vi "test robot move.vi"() -> ()   [LabVIEW 2018]
panel:
  in  "stop":bool
  in  "stop 3":bool
  in  "stop 2":bool
  out "Battery Voltage Output":u16
  in  "speed":i32
  in  "distance":dbl
  in  "Enum":enum16{"forward", "backward", "left", "right"}(ring)
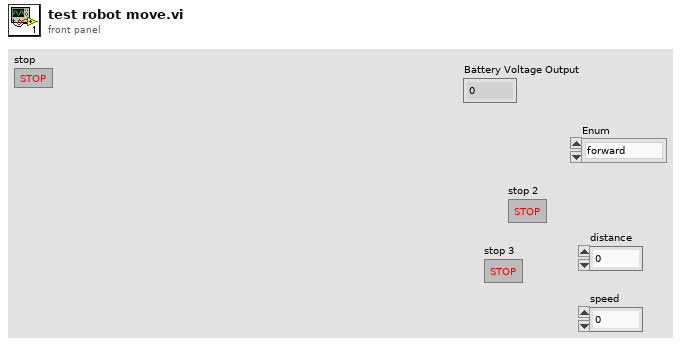
[diagram p1: front panel]
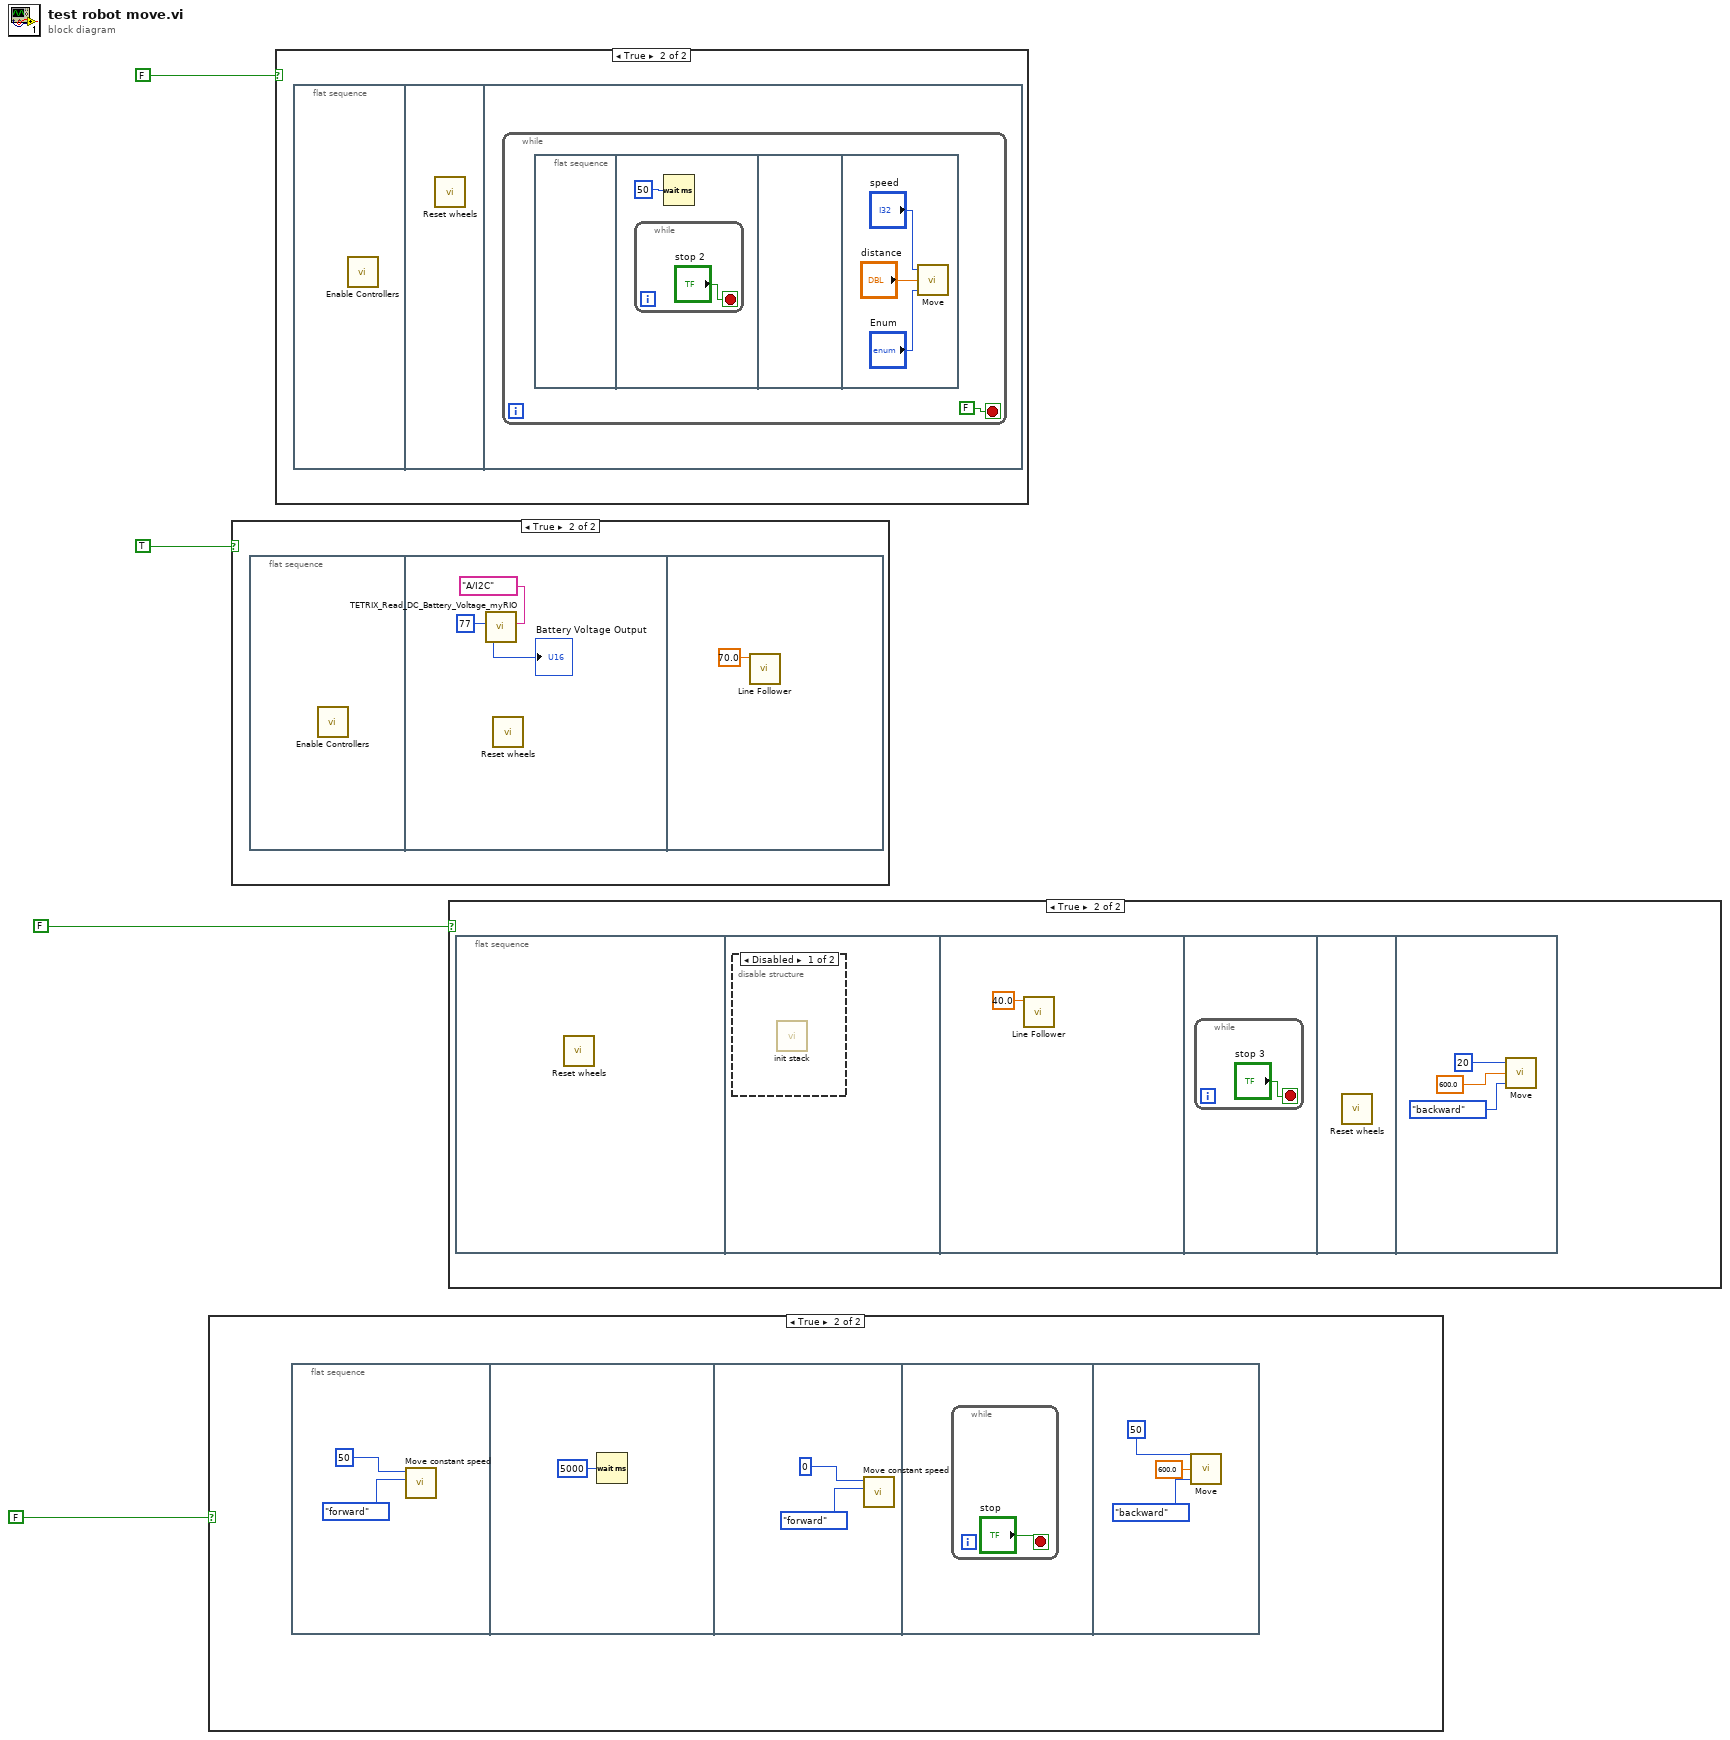
[diagram p0: block diagram]
diagram:
  n1 = case shown="True" FALSE {
    frame False {
    }
    frame True {
      n2 = flat-sequence {
        frame #0 {
          n3 = call "Move constant speed.vi"("Enum"=enum16{"forward", "backward", "left", "right"}."forward", "speed"=50) -> ()  [unwired: 10 in]
        }
        frame #1 {
          n4 = Wait (ms)(milliseconds to wait=u32 5000) -> ()  [unwired: 1 out]
        }
        frame #2 {
          n5 = call "Move constant speed.vi"("Enum"=enum16{"forward", "backward", "left", "right"}."forward", "speed"=0) -> ()  [unwired: 10 in]
        }
        frame #3 {
          n6 = while {
            stop <- "stop" stop-if-true
          }
        }
        frame #4 {
          n7 = call "Move.vi"("Enum"=enum16{"forward", "backward", "left", "right"}."backward", "distance"=600.0, "speed"=50) -> ()  [unwired: 1 in]
        }
      }
    }
  }
  n8 = case shown="True" TRUE {
    frame False {
    }
    frame True {
      n9 = flat-sequence {
        frame #0 {
          n10 = call "Enable Controllers.vi"() -> ()  [unwired: 12 in]
        }
        frame #1 {
          n11 = call <vilib>:"TETRIX_Read_DC_Battery_Voltage_myRIO.vi"("myRIO MXP Port A/B"=tag "A/I2C", "Controller ID#  (I2C Address)"=u8 77) -> ("Battery Voltage Output"=→"Battery Voltage Output":u16)  [unwired: 4 in, 1 out]
          n12 = call "Reset wheels.vi"() -> ()  [unwired: 12 in]
        }
        frame #2 {
          n13 = call "Line Follower.vi"("speed"=70.0) -> ()  [unwired: 11 in]
        }
      }
    }
  }
  n14 = case shown="True" FALSE {
    frame False {
    }
    frame True {
      n15 = flat-sequence {
        frame #0 {
          n16 = call "Enable Controllers.vi"() -> ()  [unwired: 12 in]
        }
        frame #1 {
          n17 = call "Reset wheels.vi"() -> ()  [unwired: 12 in]
        }
        frame #2 {
          n18 = while {
            stop <- FALSE stop-if-true
            n19 = flat-sequence {
              frame #0 {
              }
              frame #1 {
                n20 = while {
                  stop <- "stop 2" stop-if-true
                }
                n21 = Wait (ms)(milliseconds to wait=u32 50) -> ()  [unwired: 1 out]
              }
              frame #2 {
              }
              frame #3 {
                n22 = call "Move.vi"("Enum"="Enum", "distance"="distance", "speed"="speed") -> ()  [unwired: 1 in]
              }
            }
          }
        }
      }
    }
  }
  n23 = case shown="True" FALSE {
    frame False {
    }
    frame True {
      n24 = flat-sequence {
        frame #0 {
          n25 = call "Reset wheels.vi"() -> ()  [unwired: 12 in]
        }
        frame #1 {
          n26 = disable-structure shown="Disabled" {
            frame Disabled {
              n27 = call "init stack.vi"() -> ()  [unwired: 12 in]
            }
            frame Enabled {
            }
          }
        }
        frame #2 {
          n28 = call "Line Follower.vi"("speed"=40.0) -> ()  [unwired: 11 in]
        }
        frame #3 {
          n29 = while {
            stop <- "stop 3" stop-if-true
          }
        }
        frame #4 {
          n30 = call "Reset wheels.vi"() -> ()  [unwired: 12 in]
        }
        frame #5 {
          n31 = call "Move.vi"("Enum"=enum16{"forward", "backward", "left", "right"}."backward", "distance"=600.0, "speed"=20) -> ()  [unwired: 1 in]
        }
      }
    }
  }
